vi "rx_plot_iq.vi"(8 "error in":errorcluster, 11 "Received IQ\nwaveform":cluster{"t0":dbl, "dt":dbl, "Y":cdb[]} {"Y" format="%.2g"; "dt" format="%.2g"; "t0" format="%.2g"}) -> (0 "error out":errorcluster, 2 "Q component":waveform(dbl), 3 "I component":waveform(dbl))   [LabVIEW 2012, in "gds_hw_config.lvlib"]
uses:
  gds_hw_config.lvlib
  <vilib>/addons/Modulation/niAMT.lvlib
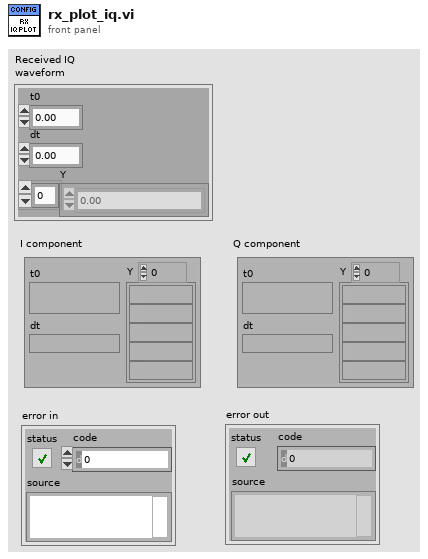
[diagram p1: front panel]
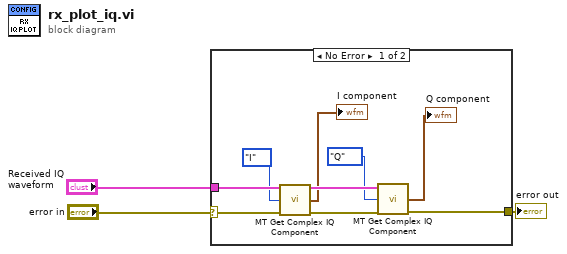
[diagram p0: block diagram]
diagram:
  n1 = case shown="No Error" "error in" {
    selector: "error in" -> [w11 w13]
    tunnel: "Received IQ\nwaveform" -> [w12 _]
    tunnel: [w8 w13] -> w1
    frame No Error {
      n2 = call <vilib>:"MT Get Complex IQ Component.vi"("IQ data (complex) in"=w12, "component choice"=enum16{"I", "Q", "Magnitude", "Phase"}."I", "error in (no error)"=w11) -> ("IQ data (complex) out"=w10:cluster{"t0":dbl, "dt":dbl, "Y":cdb[]}, "CE component"=→"I component":waveform(dbl), "error out"=w9:errorcluster)  [unwired: 10 in]
      n3 = call <vilib>:"MT Get Complex IQ Component.vi"("IQ data (complex) in"=w10, "component choice"=enum16{"I", "Q", "Magnitude", "Phase"}."Q", "error in (no error)"=w9) -> ("CE component"=→"Q component":waveform(dbl), "error out"=w8:errorcluster)  [unwired: 10 in, 1 out]
    }
    frame Error {
    }
  }
  "error out" <- w1
